vi "Main2.vi"() -> ()   [LabVIEW 2009]
uses:
  Control 3.ctl
  Global 3.vi
  <vilib>/Utility/inputDevices.llb/keyboardAcquire.vi
panel:
  out "逻辑或":bool
  in  "停止":bool
  out "字符串":string
  out "keyType 3":i32
  out "score":dbl
  out "lever":dbl
  in  "Boolean":bool=TRUE
  in  "Numeric":dbl
  out "Array":T1[][](array[typedef])
  # "贪   吃   蛇   游   戏"
  # "评语"
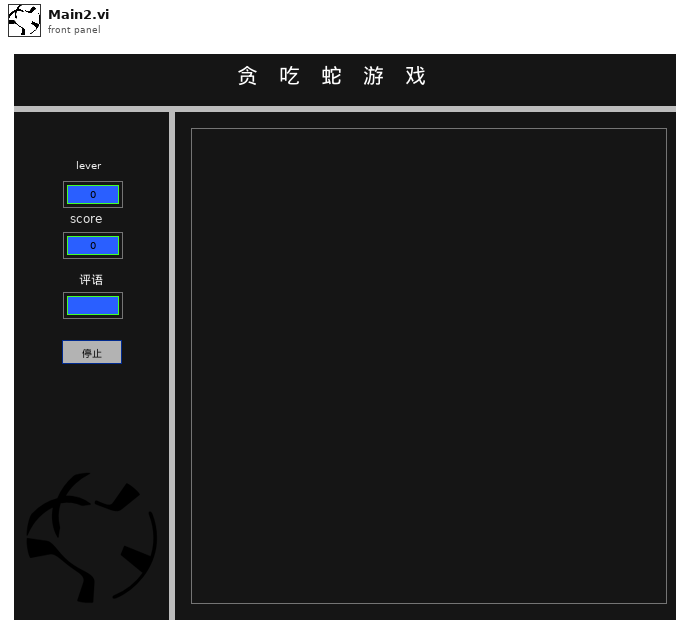
[diagram p1: front panel]
types:
  T1 = typedef "Control 3.ctl" = bool
  T2 = enum16{"0", "1", "2", "3", "4", "5", "6", "7", "8", "9", "A", "B", "C", "D", "E", "F", "G", "H", "I", "J", "K", "L", "M", "N", "O", "P", "Q", "R", "S", "T", "U", "V", "W", "X", "Y", "Z", "F1", "F2", "F3", "F4", "F5", "F6", "F7", "F8", "F9", "F10", "F11", "F12", "F13", "F14", "F15", "ADD", "BACK", "BACKSLASH", "CAPITAL", "COMMA", "DECIMAL", "DELETE", "DIVIDE", "DOWN", "END", "EQUALS", "ESCAPE", "GRAVE (`)", "HOME", "INSERT", "LBRACKET", "LCONTROL", "LEFT", "L ALT", "LSHIFT", "LWIN", "MINUS", "MULTIPLY", "NEXT", "NUMLOCK", "NUMPAD_0", "NUMPAD_1", "NUMPAD_2", "NUMPAD_3", "NUMPAD_4", "NUMPAD_5", "NUMPAD_6", "NUMPAD_7", "NUMPAD_8", "NUMPAD_9", "PAUSE", "PERIOD", "PRIOR (PG UP)", "RBRACKET", "RCONTROL", "RETURN", "RIGHT", "R ALT", "RSHIFT", "RWIN", "SCROLL", "SEMICOLON", "SLASH", "SPACE", "SUBTRACT", "TAB", "UP", "ENTER (num pad)", "' (quote)"}[]
  T3 = enum16{"0", "1", "2", "3", "4", "5", "6", "7", "8", "9", "A", "B", "C", "D", "E", "F", "G", "H", "I", "J", "K", "L", "M", "N", "O", "P", "Q", "R", "S", "T", "U", "V", "W", "X", "Y", "Z", "F1", "F2", "F3", "F4", "F5", "F6", "F7", "F8", "F9", "F10", "F11", "F12", "F13", "F14", "F15", "ADD", "BACK", "BACKSLASH", "CAPITAL", "COMMA", "DECIMAL", "DELETE", "DIVIDE", "DOWN", "END", "EQUALS", "ESCAPE", "GRAVE (`)", "HOME", "INSERT", "LBRACKET", "LCONTROL", "LEFT", "L ALT", "LSHIFT", "LWIN", "MINUS", "MULTIPLY", "NEXT", "NUMLOCK", "NUMPAD_0", "NUMPAD_1", "NUMPAD_2", "NUMPAD_3", "NUMPAD_4", "NUMPAD_5", "NUMPAD_6", "NUMPAD_7", "NUMPAD_8", "NUMPAD_9", "PAUSE", "PERIOD", "PRIOR (PG UP)", "RBRACKET", "RCONTROL", "RETURN", "RIGHT", "R ALT", "RSHIFT", "RWIN", "SCROLL", "SEMICOLON", "SLASH", "SPACE", "SUBTRACT", "TAB", "UP", "ENTER (num pad)", "' (quote)"}
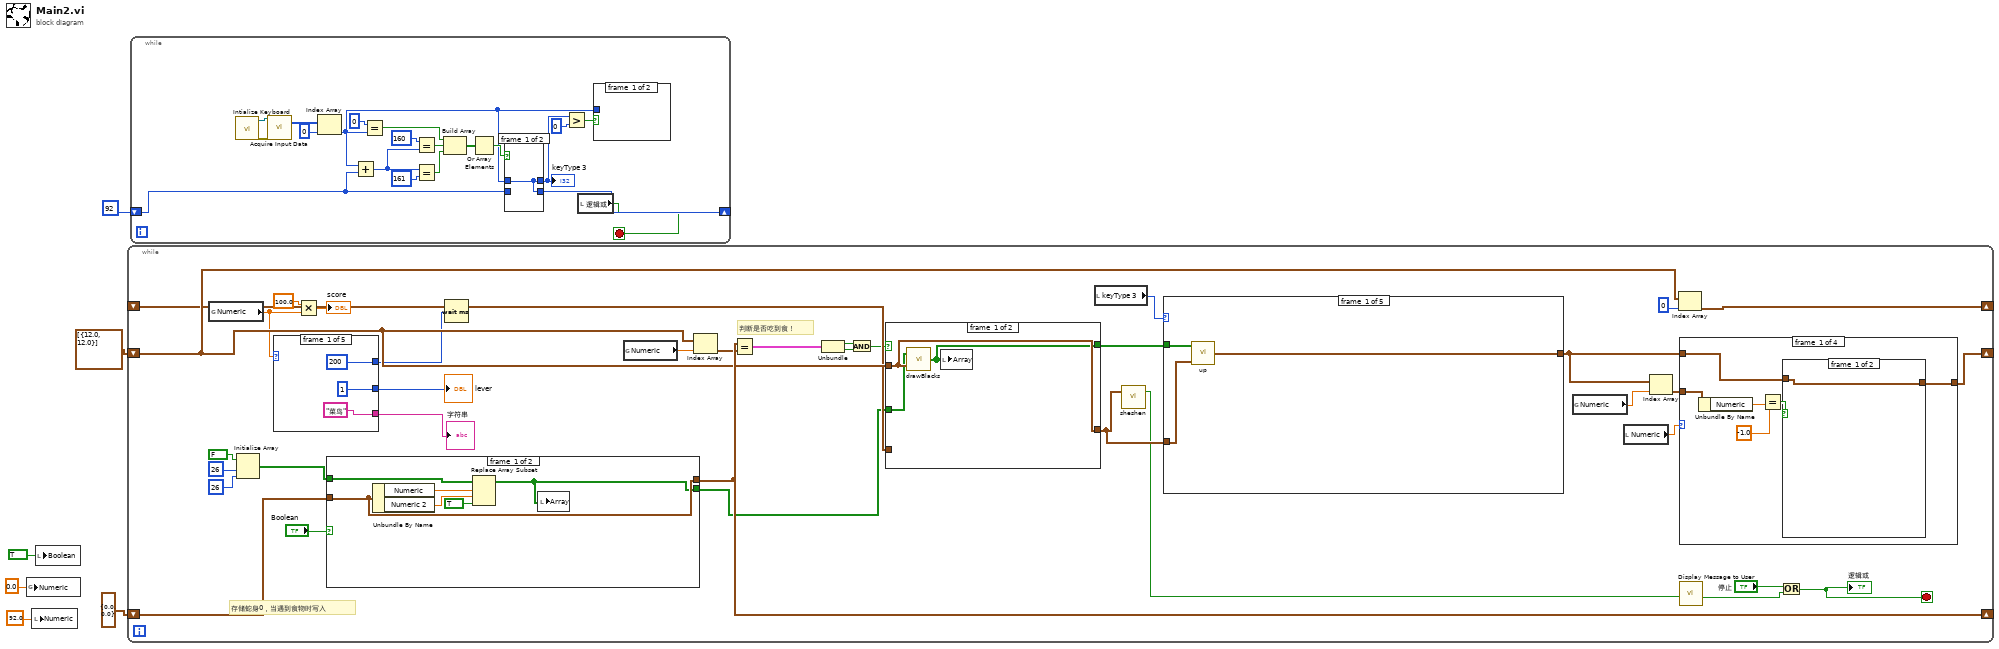
[diagram p0: block diagram]
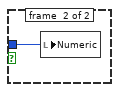
[diagram p2: hidden frame]
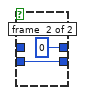
[diagram p3: hidden frame]
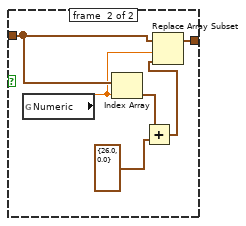
[diagram p4: hidden frame]
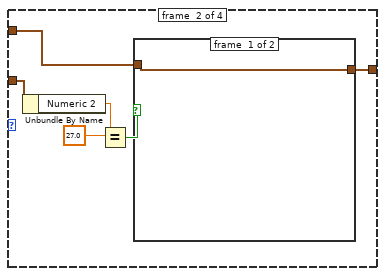
[diagram p5: hidden frame]
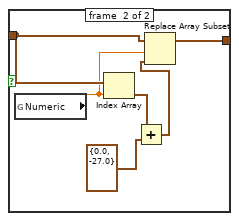
[diagram p6: hidden frame]
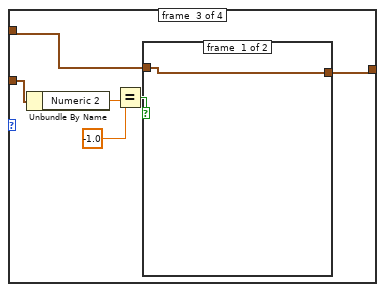
[diagram p7: hidden frame]
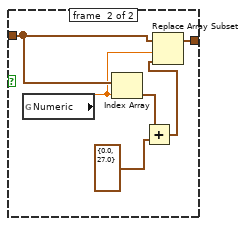
[diagram p8: hidden frame]
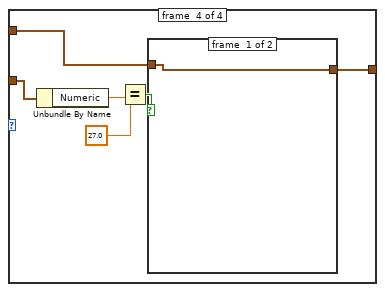
[diagram p9: hidden frame]
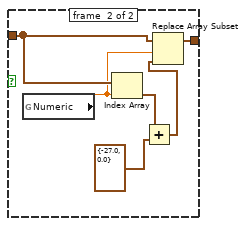
[diagram p10: hidden frame]
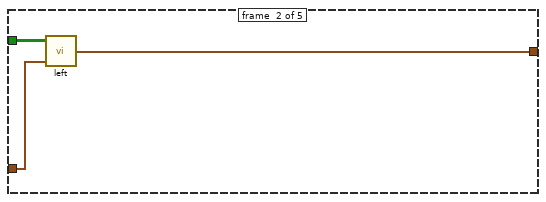
[diagram p11: hidden frame]
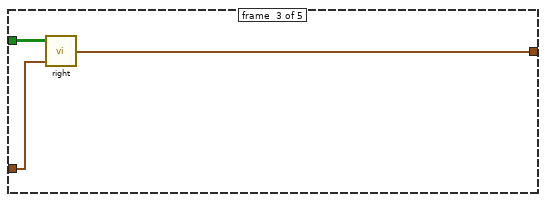
[diagram p12: hidden frame]
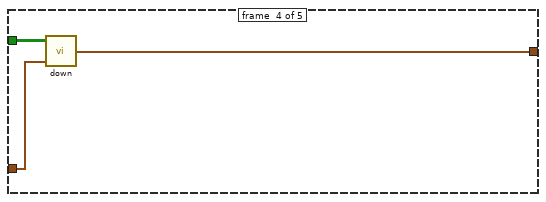
[diagram p13: hidden frame]
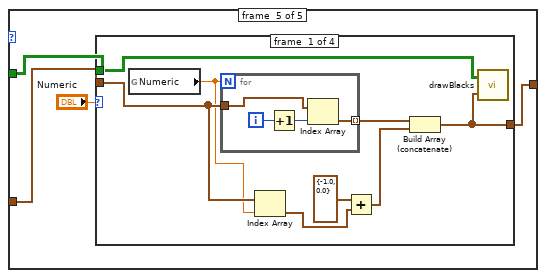
[diagram p14: hidden frame]
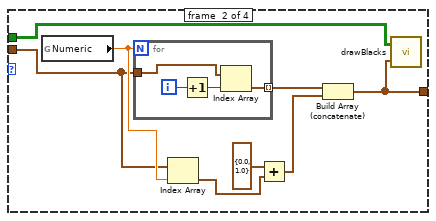
[diagram p15: hidden frame]
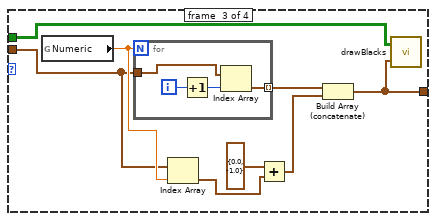
[diagram p16: hidden frame]
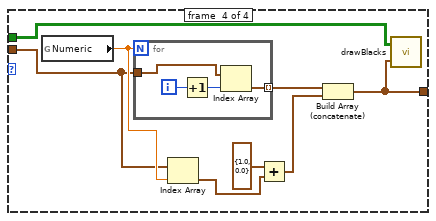
[diagram p17: hidden frame]
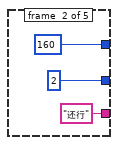
[diagram p18: hidden frame]
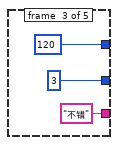
[diagram p19: hidden frame]
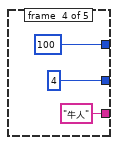
[diagram p20: hidden frame]
diagram:
  n1 = global write "Global 3.vi" "Numeric"(0.0 ("Numeric")) -> ()
  n2 = local write "Numeric"(92.0 ("Numeric")) -> ()
  n3 = local write "Boolean"(TRUE ("Boolean")) -> ()
  n4 = while {
    shift-right: [w37] -> _
    shift-left: cluster{"Numeric":dbl, "Numeric 2":dbl}[] [{"Numeric"=12.0, "Numeric 2"=12.0}] ("Array 2") -> [w40]
    shift-right: [w41] -> _
    shift-left: cluster{"Numeric":dbl, "Numeric 2":dbl} {"Numeric"=0.0, "Numeric 2"=0.0} ("x") -> [w42]
    shift-right: [w39] -> _
    shift-left: _ -> [w38]
    stop <- w36 stop-if-true
    # "存储蛇身0，当遇到食物时写入"
    # "判断是否吃到食！"
    n5 = global read "Global 3.vi" "Numeric"() -> (w20:dbl)
    n6 = Initialize Array(FALSE, 26 ("dimension size"), 26 ("dimension size")) -> (w31:bool[][])
    n7 = case shown="11, 默认" w20 {
      tunnel: [200 160 120 100 80] -> w17
      tunnel: [1 2 3 4 5] -> w22
      tunnel: ["菜鸟" "还行" "不错" "牛人" "神人"] -> w10
      frame #0 {
      }
      frame #1 {
      }
      frame #2 {
      }
      frame #3 {
      }
      frame #4 {
        # "等级！"
      }
    }
    "lever" <- w22
    "字符串" <- w10
    n8 = Multiply(x=100.0, y=w20) -> (x*y=→"score":dbl)
    n9 = case shown="真" "Boolean" {
      tunnel: [w186 w197] -> w23
      tunnel: w31 -> [w191 w196]
      tunnel: [w190 w192] -> w41
      tunnel: w42 -> [w190 _]
      frame #0 {
        n10 = Unbundle By Name(w190) -> ("Numeric"=w189:dbl, "Numeric 2"=w188:dbl)
        n11 = Replace Array Subset(array=w191, new element=T1 TRUE ("new element/subarray"), index (row)=w189, index (col)=w188) -> (w186:bool[][])
        n12 = local write "Array"(w186) -> ()
      }
      frame #1 {
        # "随机生成食物！"
        n13 = local write "Boolean"(FALSE ("Boolean")) -> ()
        n14 = Random Number (0-1)() -> (number: 0 to 1=w202:dbl)
        n15 = Random Number (0-1)() -> (number: 0 to 1=w203:dbl)
        n16 = Multiply(x=w203, y=10.0) -> (x*y=w200:dbl)
        n17 = Multiply(x=w202, y=24.0) -> (x*y=w204:dbl)
        n18 = Round To Nearest(number=w200) -> (nearest integer value=w194:dbl)
        n19 = Round To Nearest(number=w204) -> (nearest integer value=w193:dbl)
        n20 = Replace Array Subset(array=w196, new element=T1 TRUE ("new element/subarray"), index (row)=w194, index (col)=w193) -> (w197:bool[][])
        "Array" <- w197
        n21 = Bundle(w194, w193) -> (w192:cluster{dbl, dbl})  [unwired: 1 in]
      }
    }
    n22 = Wait (ms)(milliseconds to wait=w17) -> ()  [unwired: 1 out]
    n23 = global read "Global 3.vi" "Numeric"() -> (w29:dbl)
    n24 = Index Array(array=w40, index=w29) -> (element=w24:cluster{"Numeric":dbl, "Numeric 2":dbl})
    n25 = Equal?(x=w41, y=w24) -> (x = y?=w28:cluster{"Numeric":bool, "Numeric 2":bool})
    n26 = Unbundle(w28) -> ("Numeric"=w27:bool, "Numeric 2"=w26:bool)
    n27 = And(x=w27, y=w26) -> (x .and. y?=w25:bool)
    n28 = case shown="假" w25 {
      tunnel: w40 -> [w176 w183]
      tunnel: [w176 w182] -> w15
      tunnel: w23 -> [w175 w181]
      tunnel: [w174 w179] -> w35
      tunnel: w38 -> [_ w178]
      frame #0 {
        n29 = call "drawBlacks.vi"("Array 2"=w176, "Array 3"=w175) -> ("Array"=w174:bool[][])
        n30 = local write "Array"(w174) -> ()
      }
      frame #1 {
        n31 = global read "Global 3.vi" "Numeric"() -> (w185:dbl)
        n32 = local write "Boolean"(TRUE ("Boolean")) -> ()
        n33 = Insert Into Array(array=w183, index=0 ("索引"), new element=w178) -> (w182:cluster{"Numeric":dbl, "Numeric 2":dbl}[])
        n34 = Increment(x=w185) -> (x+1=w184:dbl)
        n35 = call "drawBlacks.vi"("Array 2"=w182, "Array 3"=w181) -> ("Array"=w179:bool[][])
        n36 = global write "Global 3.vi" "Numeric"(w184) -> ()
        n37 = local write "Array"(w179) -> ()
      }
    }
    n38 = local read "keyType 3"() -> (w18:i32)
    n39 = call "sheshen.vi"("数组"=w15) -> ("逻辑或"=w9:bool)  [unwired: 2 in]
    n40 = case shown="0, 默认" w18 {
      tunnel: w15 -> [w96 w99 w102 w105 w110]
      tunnel: w35 -> [w97 w100 w101 w106 w109]
      tunnel: [w95 w98 w103 w104 w108] -> w11
      frame #0 {
        n41 = call "up.vi"("Array 2"=w96, "initialized array"=w97) -> ("appended array"=w95:cluster{"Numeric":dbl, "Numeric 2":dbl}[])  [unwired: 1 in, 2 out]
      }
      frame #1 {
        n42 = call "left.vi"("Array 2"=w99, "initialized array"=w100) -> ("appended array"=w98:cluster{"Numeric":dbl, "Numeric 2":dbl}[])  [unwired: 1 in, 2 out]
      }
      frame #2 {
        n43 = call "right.vi"("Array 2"=w102, "initialized array"=w101) -> ("appended array"=w103:cluster{"Numeric":dbl, "Numeric 2":dbl}[])  [unwired: 1 in, 2 out]
      }
      frame #3 {
        n44 = call "down.vi"("Array 2"=w105, "initialized array"=w106) -> ("appended array"=w104:cluster{"Numeric":dbl, "Numeric 2":dbl}[])  [unwired: 1 in, 2 out]
      }
      frame #4 {
        n45 = case shown="92" "Numeric" {
          tunnel: w109 -> [w118 w130 w142 w154]
          tunnel: w110 -> [w114 w125 w137 w149]
          tunnel: [w113 w124 w136 w148] -> w108
          frame #0 {
            n46 = global read "Global 3.vi" "Numeric"() -> (w112:dbl)
            n47 = for {
              N: w112 -> [_]
              tunnel: w114 -> [w122]
              tunnel: [w119] -> w117 mode=indexing
              i -> [w121]
              n48 = Increment(x=w121) -> (x+1=w120:i32)
              n49 = Index Array(array=w122, index=w120) -> (element=w119:cluster{"Numeric":dbl, "Numeric 2":dbl})
            }
            n50 = Index Array(array=w114, index=w112) -> (element=w115:cluster{"Numeric":dbl, "Numeric 2":dbl})
            n51 = Add(x=cluster{"Numeric":dbl, "Numeric 2":dbl} {"Numeric"=-1.0, "Numeric 2"=0.0}, y=w115) -> (x+y=w111:cluster{"Numeric":dbl, "Numeric 2":dbl})
            n52 = Build Array (concatenate)(w117, w111) -> (w113:cluster{"Numeric":dbl, "Numeric 2":dbl}[])
            n53 = call "drawBlacks.vi"("Array 2"=w113, "Array 3"=w118) -> ()  [unwired: 1 out]
          }
          frame #1 {
            n54 = global read "Global 3.vi" "Numeric"() -> (w126:dbl)
            n55 = for {
              N: w126 -> [_]
              tunnel: w125 -> [w134]
              tunnel: [w131] -> w129 mode=indexing
              i -> [w133]
              n56 = Increment(x=w133) -> (x+1=w132:i32)
              n57 = Index Array(array=w134, index=w132) -> (element=w131:cluster{"Numeric":dbl, "Numeric 2":dbl})
            }
            n58 = Index Array(array=w125, index=w126) -> (element=w127:cluster{"Numeric":dbl, "Numeric 2":dbl})
            n59 = Add(x=cluster{"Numeric":dbl, "Numeric 2":dbl} {"Numeric"=0.0, "Numeric 2"=1.0}, y=w127) -> (x+y=w123:cluster{"Numeric":dbl, "Numeric 2":dbl})
            n60 = Build Array (concatenate)(w129, w123) -> (w124:cluster{"Numeric":dbl, "Numeric 2":dbl}[])
            n61 = call "drawBlacks.vi"("Array 2"=w124, "Array 3"=w130) -> ()  [unwired: 1 out]
          }
          frame #2 {
            n62 = global read "Global 3.vi" "Numeric"() -> (w138:dbl)
            n63 = for {
              N: w138 -> [_]
              tunnel: w137 -> [w146]
              tunnel: [w143] -> w141 mode=indexing
              i -> [w145]
              n64 = Increment(x=w145) -> (x+1=w144:i32)
              n65 = Index Array(array=w146, index=w144) -> (element=w143:cluster{"Numeric":dbl, "Numeric 2":dbl})
            }
            n66 = Index Array(array=w137, index=w138) -> (element=w139:cluster{"Numeric":dbl, "Numeric 2":dbl})
            n67 = Add(x=cluster{"Numeric":dbl, "Numeric 2":dbl} {"Numeric"=0.0, "Numeric 2"=-1.0}, y=w139) -> (x+y=w135:cluster{"Numeric":dbl, "Numeric 2":dbl})
            n68 = Build Array (concatenate)(w141, w135) -> (w136:cluster{"Numeric":dbl, "Numeric 2":dbl}[])
            n69 = call "drawBlacks.vi"("Array 2"=w136, "Array 3"=w142) -> ()  [unwired: 1 out]
          }
          frame #3 {
            n70 = global read "Global 3.vi" "Numeric"() -> (w150:dbl)
            n71 = for {
              N: w150 -> [_]
              tunnel: w149 -> [w158]
              tunnel: [w155] -> w153 mode=indexing
              i -> [w157]
              n72 = Increment(x=w157) -> (x+1=w156:i32)
              n73 = Index Array(array=w158, index=w156) -> (element=w155:cluster{"Numeric":dbl, "Numeric 2":dbl})
            }
            n74 = Index Array(array=w149, index=w150) -> (element=w151:cluster{"Numeric":dbl, "Numeric 2":dbl})
            n75 = Add(x=cluster{"Numeric":dbl, "Numeric 2":dbl} {"Numeric"=1.0, "Numeric 2"=0.0}, y=w151) -> (x+y=w147:cluster{"Numeric":dbl, "Numeric 2":dbl})
            n76 = Build Array (concatenate)(w153, w147) -> (w148:cluster{"Numeric":dbl, "Numeric 2":dbl}[])
            n77 = call "drawBlacks.vi"("Array 2"=w148, "Array 3"=w154) -> ()  [unwired: 1 out]
          }
        }
      }
    }
    n78 = global read "Global 3.vi" "Numeric"() -> (w14:dbl)
    n79 = local read "Numeric"() -> (w13:dbl)
    n80 = Index Array(array=w11, index=w14) -> (element=w12:cluster{"Numeric":dbl, "Numeric 2":dbl})
    n81 = Index Array(array=w40, index=0 ("索引")) -> (element=w39:cluster{"Numeric":dbl, "Numeric 2":dbl})
    n82 = case shown="92" w13 {
      tunnel: w12 -> [w48 w56 w70 w83]
      tunnel: w11 -> [w44 w57 w71 w84]
      tunnel: [w43 w58 w69 w82] -> w37
      frame #0 {
        n83 = Unbundle By Name(w48) -> ("Numeric"=w47:dbl)
        n84 = Equal?(x=-1.0, y=w47) -> (x = y?=w45:bool)
        n85 = case shown="真" w45 {
          tunnel: w44 -> [w49 w53]
          tunnel: [w49 w50] -> w43
          frame #0 {
          }
          frame #1 {
            n86 = global read "Global 3.vi" "Numeric"() -> (w52:dbl)
            n87 = Index Array(array=w53, index=w52) -> (element=w55:cluster{"Numeric":dbl, "Numeric 2":dbl})
            n88 = Add(x=w55, y=cluster{"Numeric":dbl, "Numeric 2":dbl} {"Numeric"=26.0, "Numeric 2"=0.0} ("新元素/子数组")) -> (x+y=w51:cluster{"Numeric":dbl, "Numeric 2":dbl})
            n89 = Replace Array Subset(array=w53, new element=w51, index=w52) -> (w50:cluster{"Numeric":dbl, "Numeric 2":dbl}[])
          }
        }
      }
      frame #1 {
        n90 = Unbundle By Name(w56) -> ("Numeric 2"=w61:dbl)
        n91 = Equal?(x=27.0, y=w61) -> (x = y?=w59:bool)
        n92 = case shown="真" w59 {
          tunnel: w57 -> [w62 w66]
          tunnel: [w62 w63] -> w58
          frame #0 {
          }
          frame #1 {
            n93 = global read "Global 3.vi" "Numeric"() -> (w65:dbl)
            n94 = Index Array(array=w66, index=w65) -> (element=w68:cluster{"Numeric":dbl, "Numeric 2":dbl})
            n95 = Add(x=w68, y=cluster{"Numeric":dbl, "Numeric 2":dbl} {"Numeric"=0.0, "Numeric 2"=-27.0} ("新元素/子数组")) -> (x+y=w64:cluster{"Numeric":dbl, "Numeric 2":dbl})
            n96 = Replace Array Subset(array=w66, new element=w64, index=w65) -> (w63:cluster{"Numeric":dbl, "Numeric 2":dbl}[])
          }
        }
      }
      frame #2 {
        n97 = Unbundle By Name(w70) -> ("Numeric 2"=w74:dbl)
        n98 = Equal?(x=-1.0, y=w74) -> (x = y?=w72:bool)
        n99 = case shown="真" w72 {
          tunnel: w71 -> [w75 w79]
          tunnel: [w75 w76] -> w69
          frame #0 {
          }
          frame #1 {
            n100 = global read "Global 3.vi" "Numeric"() -> (w78:dbl)
            n101 = Index Array(array=w79, index=w78) -> (element=w81:cluster{"Numeric":dbl, "Numeric 2":dbl})
            n102 = Add(x=w81, y=cluster{"Numeric":dbl, "Numeric 2":dbl} {"Numeric"=0.0, "Numeric 2"=27.0} ("新元素/子数组")) -> (x+y=w77:cluster{"Numeric":dbl, "Numeric 2":dbl})
            n103 = Replace Array Subset(array=w79, new element=w77, index=w78) -> (w76:cluster{"Numeric":dbl, "Numeric 2":dbl}[])
          }
        }
      }
      frame #3 {
        n104 = Unbundle By Name(w83) -> ("Numeric"=w87:dbl)
        n105 = Equal?(x=27.0, y=w87) -> (x = y?=w85:bool)
        n106 = case shown="真" w85 {
          tunnel: w84 -> [w88 w92]
          tunnel: [w88 w89] -> w82
          frame #0 {
          }
          frame #1 {
            n107 = global read "Global 3.vi" "Numeric"() -> (w91:dbl)
            n108 = Index Array(array=w92, index=w91) -> (element=w94:cluster{"Numeric":dbl, "Numeric 2":dbl})
            n109 = Add(x=w94, y=cluster{"Numeric":dbl, "Numeric 2":dbl} {"Numeric"=-27.0, "Numeric 2"=0.0} ("新元素/子数组")) -> (x+y=w90:cluster{"Numeric":dbl, "Numeric 2":dbl})
            n110 = Replace Array Subset(array=w92, new element=w90, index=w91) -> (w89:cluster{"Numeric":dbl, "Numeric 2":dbl}[])
          }
        }
      }
    }
    n111 = call "Display Message to User"("Enable"=w9) -> ("OK"=w7:bool)  [unwired: 9 in, 1 out]
    n112 = Or(x="停止", y=w7) -> (x .or. y?=w36:bool)
    "逻辑或" <- w36
  }
  n113 = while {
    shift-right: [w223] -> _
    shift-left: 92 -> [w224]
    stop <- w222 stop-if-true
    n114 = call <vilib>:"Intialize Keyboard.vi"() -> ("error out"=w220:errorcluster, "device ID"=w221:refnum<k1>)  [unwired: 10 in]
    n115 = call-poly <vilib>:"Acquire Input Data.vi"("device ID"=w221, "error in (no error)"=w220) -> ("keys pressed"=w218:T2)  [unwired: 15 in, 2 out]
    n116 = Index Array(array=w218, index=0 ("索引")) -> (element=w205:T3)
    n117 = Add(x=w205, y=w224) -> (x+y=w216:i32)
    n118 = Equal?(x=0, y=w205) -> (x = y?=w213:bool)
    n119 = Equal?(x=160, y=w216) -> (x = y?=w212:bool)
    n120 = Equal?(x=w216, y=161) -> (x = y?=w211:bool)
    n121 = Build Array(w213, w212, w211) -> (w210:bool[])
    n122 = Or Array Elements(Boolean array=w210) -> (logical OR=w209:bool)
    n123 = case shown="真" w209 {
      tunnel: w205 -> [w226 _]
      tunnel: [w226 0] -> w206
      tunnel: w224 -> [_ w227]
      tunnel: [w226 w227] -> w223
      frame #0 {
      }
      frame #1 {
      }
    }
    "keyType 3" <- w206
    n124 = Greater?(x=w206, y=0) -> (0:w207:bool)
    n125 = local read "逻辑或"() -> (w222:bool)
    n126 = case shown="真" w207 {
      tunnel: w205 -> [_ w225]
      frame #0 {
      }
      frame #1 {
        n127 = local write "Numeric"(w225) -> ()
      }
    }
  }
